vi "PopOpen.vi"() -> ()   [LabVIEW 2013, in "RVCLibrary_Bug2.lvclass"]
uses:
  RVCLibrary_Bug2.lvclass
  <vilib>/robotics/Navigation/shared/MapNode/AbstractDstarNode/NI_Robotics_AbstractDstarNode.lvclass
  <vilib>/robotics/Navigation/shared/Priority Queue/NI_Robotics_Priority Queue.lvclass
  <vilib>/robotics/Navigation/Anytime D Star/NI_Robotics_AnytimeDStar.lvclass
  <vilib>/robotics/Navigation/shared/MapNode/AbstractMapNode/NI_Robotics_AbstractMapNode.lvclass
  <vilib>/robotics/Navigation/shared/Priority Queue/Open List Element.ctl
panel:
  in  "RVCLibrary_Bug2 in":refnum<class "RVCLibrary_Bug2.lvclass">
  out "empty":bool
  out "open list element":T1
  out "error out 2":errorcluster
  in  "error in (no error) 2":errorcluster
  out "error out":errorcluster
  in  "error in (no error)":errorcluster
  out "node ref out":refnum<data-value>
  out "AD* out":refnum<class "NI_Robotics_AnytimeDStar.lvclass">
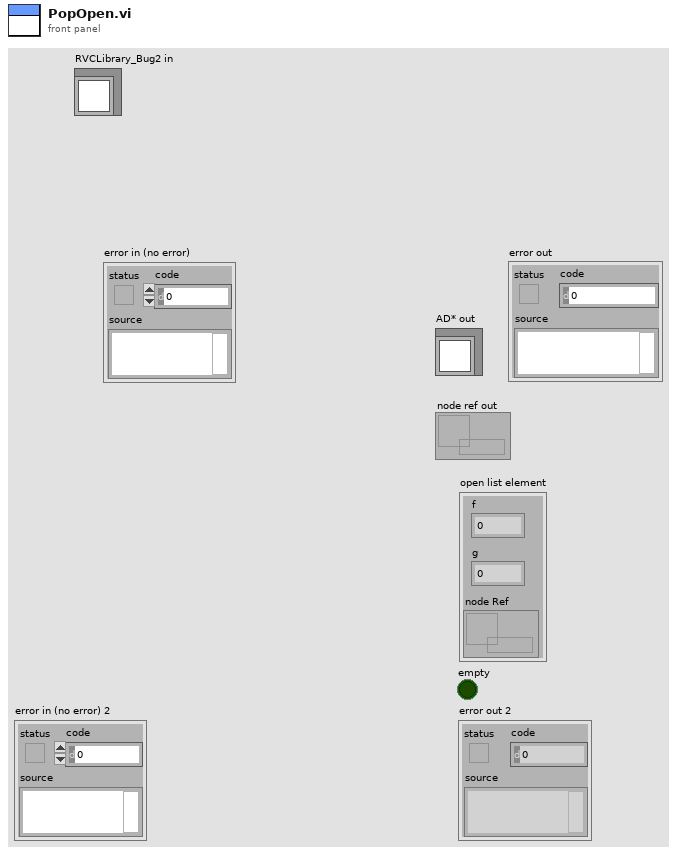
[diagram p1: front panel]
types:
  T1 = typedef "NI_Robotics_Priority Queue.lvclass/Open List Element.ctl" = cluster{"f":dbl, "g":dbl, "node Ref":refnum<data-value>}
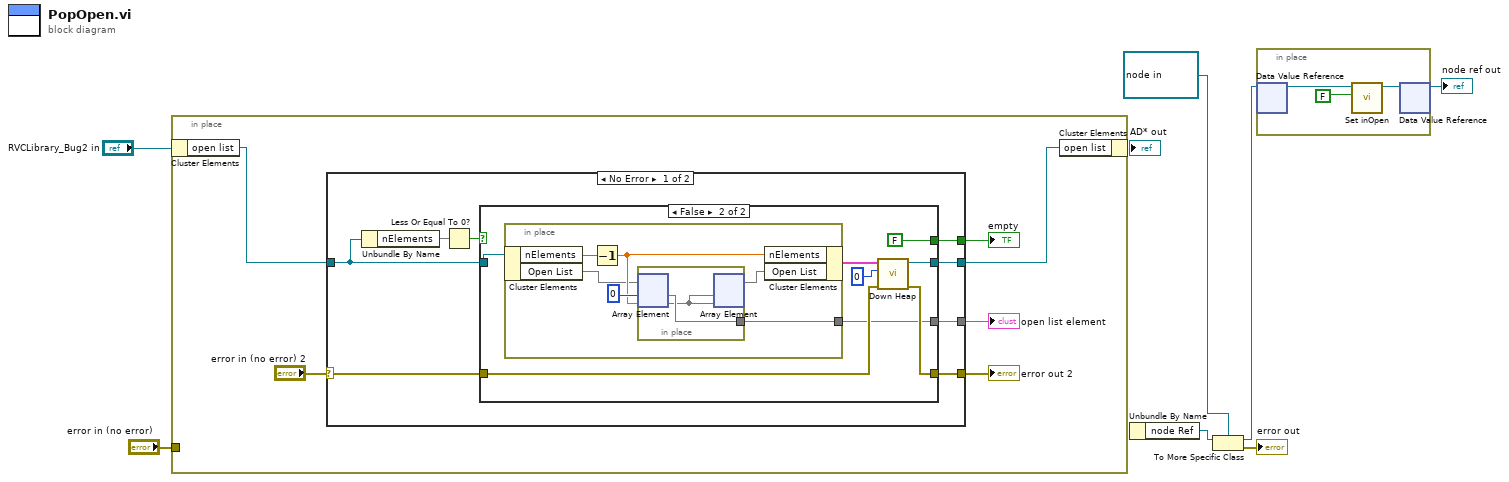
[diagram p0: block diagram]
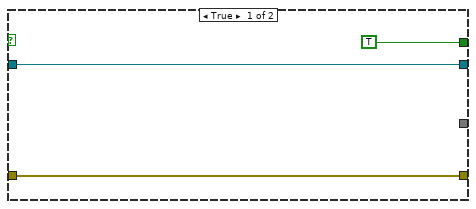
[diagram p2: hidden frame]
diagram:
  n1 = in-place {
    in-place-border: "error in (no error)" -> [_]
    n2 = in-place-cluster #1("RVCLibrary_Bug2 in") -> ("open list"=w9:refnum<class "NI_Robotics_Priority Queue.lvclass">)
    n3 = case shown="No Error" "error in (no error) 2" {
      selector: "error in (no error) 2" -> [w16 w42]
      tunnel: [w21 w42] -> w13
      tunnel: [w20 w41] -> w8
      tunnel: w9 -> [w19 w41]
      tunnel: [w18 _] -> w12
      tunnel: [w17 _] -> w11
      frame No Error {
        n4 = Unbundle By Name(w19) -> ("nElements"=w15)
        n5 = Less Or Equal To 0?(x=w15) -> (x <= 0?=w14:bool)
        n6 = case shown="False" w14 {
          tunnel: [w23 w29] -> w21
          tunnel: [w24 w31] -> w20
          tunnel: w19 -> [w24 w32]
          tunnel: w16 -> [w23 w30]
          tunnel: [_ w27] -> w18
          tunnel: [TRUE ("status") FALSE ("status")] -> w17
          frame True {
          }
          frame False {
            n7 = in-place {
              in-place-border: [w33] -> w27
              n8 = in-place-cluster #2(w32) -> ("nElements"=w38, "Open List"=w35)
              n9 = Decrement(x=w38) -> (x-1=w36:dbl)
              n10 = in-place {
                in-place-border: [w40] -> w33
                n11 = in-place-array #3(w35, 0 ("index"), w36) -> (w40, w39)
                n12 = in-place-array #3(w39, w39) -> (w34)  [unwired: 2 out]
              }
              n13 = in-place-cluster #2("nElements"=w36, "Open List"=w34) -> (w25:cluster{})
            }
            n14 = call <vilib>:"Down Heap.vi"("error in (no error)"=w30, "index"=0, "Astar Open List in"=w25) -> ("error out"=w29:errorcluster, "Astar Open List out"=w31:refnum<class "NI_Robotics_Priority Queue.lvclass">)  [unwired: 7 out]
          }
        }
      }
      frame Error {
      }
    }
    "error out 2" <- w13
    "open list element" <- w12
    "empty" <- w11
    n15 = in-place-cluster #1("open list"=w8) -> ()  [unwired: 1 out]
  }
  n16 = Unbundle By Name() -> ("node Ref"=w7:refnum<data-value>)  [unwired: 1 in]
  n17 = To More Specific Class(target class=refnum<data-value> refnum ("node ref out"), reference=w7) -> (specific class reference=w6:refnum<data-value>, error out=→"error out":errorcluster)  [unwired: 1 in]
  n18 = in-place {
    n19 = in-place-dvr #4(w6) -> (w44:refnum<class "NI_Robotics_AbstractDstarNode.lvclass">)  [unwired: 1 out]
    n20 = call <vilib>:"Set inOpen.vi"("inOpen"=FALSE, "AbstractDstarNode in"=w44) -> ("AbstractDstarNode out"=w43:refnum<class "NI_Robotics_AbstractDstarNode.lvclass">)  [unwired: 8 in, 1 out]
    n21 = in-place-dvr #4(w43) -> (→"node ref out":refnum<data-value>)  [unwired: 1 out]
  }
